vi "Gen_ISH_data.vi"(5 "Исходные данные":T1) -> (2 "Исходные tbl":string[][](table))   [LabVIEW 2023, in "Registration.lvlib"]
uses:
  Registration.lvlib
  Initial Data/InitalData Type.ctl
  Initial Data/Initial Data.lvlib
panel:
  # "Образец"
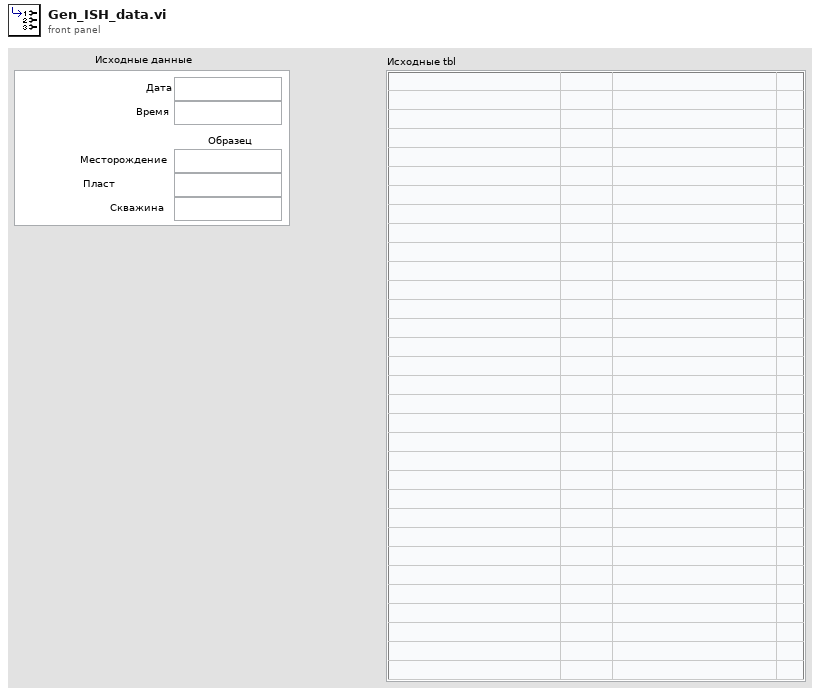
[diagram p1: front panel]
types:
  T1 = typedef "Initial Data.lvlib/InitalData Type.ctl" = cluster{"Дата":string, "Время":string, "Месторождение":string, "Пласт":string, "Скважина":string}
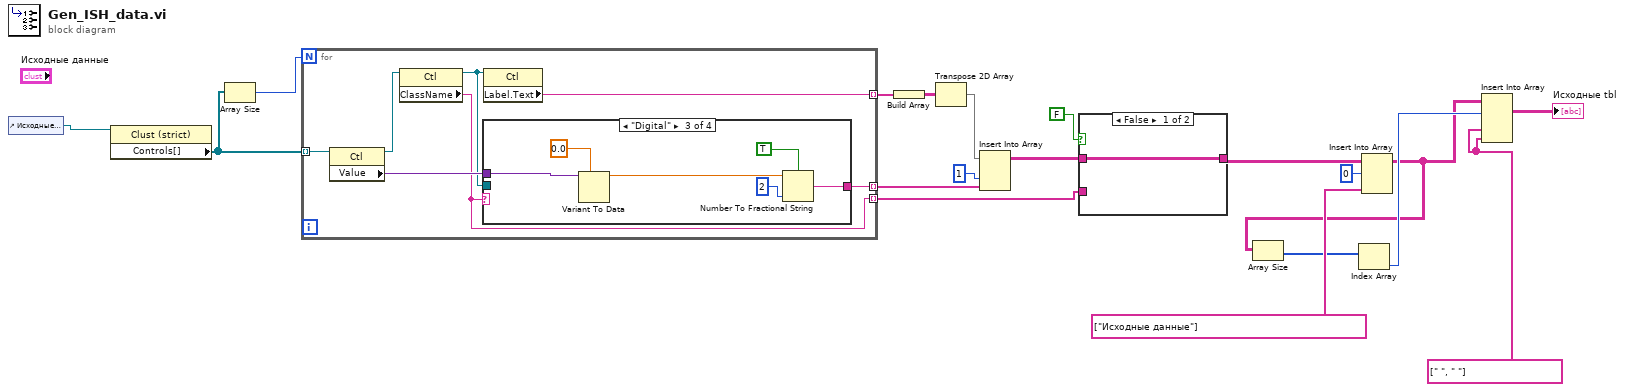
[diagram p0: block diagram]
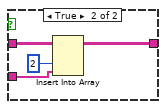
[diagram p2: hidden frame]
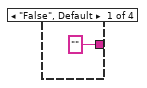
[diagram p3: hidden frame]
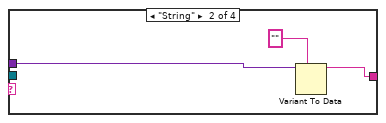
[diagram p4: hidden frame]
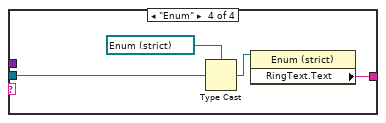
[diagram p5: hidden frame]
diagram:
  w4 = string[] [" ", " "] ("new element/subarray")
  n1 = control-ref of="Исходные данные"() -> (w3:refnum<vi>)
  n2 = property class="Clust (strict)"(reference=w3) -> ("Controls[]"=w2:refnum<vi>[])  [unwired: 1 in, 2 out]
  n3 = Array Size(array=w2) -> (size(s)=w1:i32)
  n4 = for {
    N: w1 -> [_]
    tunnel: [w23] -> w18 mode=indexing
    tunnel: w2 -> [w24] mode=indexing
    tunnel: [w22] -> w17 mode=indexing
    tunnel: [w21] -> w13 mode=indexing
    n5 = property class="Ctl"(reference=w24) -> (reference out=w25:refnum<vi>, "Value"=w26:variant)  [unwired: 1 in, 1 out]
    n6 = property class="Ctl"(reference=w25) -> (reference out=w20:refnum<vi>, "ClassName"=w21:string)  [unwired: 1 in, 1 out]
    n7 = case shown="\"Digital\"" w21 {
      tunnel: w26 -> [_ w29 w36 _]
      tunnel: ["" w28 w33 w38] -> w23
      tunnel: w20 -> [_ _ _ w40]
      frame "False", Default {
      }
      frame "String" {
        n8 = Variant To Data(type="", Variant=w29) -> (data=w28:string)  [unwired: 1 in, 1 out]
      }
      frame "Digital" {
        n9 = Variant To Data(type=0.0, Variant=w36) -> (data=w34:dbl)  [unwired: 1 in, 1 out]
        n10 = Number To Fractional String(use system decimal point (T)=TRUE, number=w34, precision (6)=i16 2) -> (F-format string=w33:string)  [unwired: 1 in]
      }
      frame "Enum" {
        n11 = Type Cast(type=refnum<vi> refnum ("Enum"), x=w40) -> (*(type *) &x=w39:refnum<vi>)
        n12 = property class="Enum (strict)"(reference=w39) -> ("RingText.Text"=w38:string)  [unwired: 1 in, 2 out]
      }
    }
    n13 = property class="Ctl"(reference=w20) -> ("Label.Text"=w22:string)  [unwired: 1 in, 2 out]
  }
  n14 = Build Array(w17) -> (w16:string[][])
  n15 = Transpose 2D Array(2D array=w16) -> (transposed array=w15:string[][])
  n16 = Insert Into Array "Insert Into Array"(array=w15, index (col)=1 ("disabled index (col)"), new element=w18) -> (w14:string[][])  [unwired: 1 in]
  n17 = case shown="False" FALSE {
    tunnel: w14 -> [w41 w45]
    tunnel: w13 -> [_ w43]
    tunnel: [w41 w42] -> w9
    frame False {
    }
    frame True {
      n18 = Insert Into Array "Insert Into Array"(array=w45, index (col)=2 ("disabled index (col)"), new element=w43) -> (w42:string[][])  [unwired: 1 in]
    }
  }
  n19 = Insert Into Array "Insert Into Array"(array=w9, index (row)=0, new element=string[] ["Исходные данные"] ("new element/subarray")) -> (w5:string[][])  [unwired: 1 in]
  n20 = Array Size(array=w5) -> (size(s)=w7:i32[])
  n21 = Index Array(array=w7) -> (element=w6:i32)  [unwired: 1 in]
  n22 = Insert Into Array "Insert Into Array"(array=w5, index (row)=w6, new element #1=w4, new element #2=w4) -> (→"Исходные tbl":string[][])  [unwired: 1 in]
